vi "Software Update HCC Machine Download Status.vi"(9 "Progam Number":i32, 10 "Station Labels":string[](array[string]), 11 "File Path":path) -> (3 "Status":string)   [LabVIEW 2014]
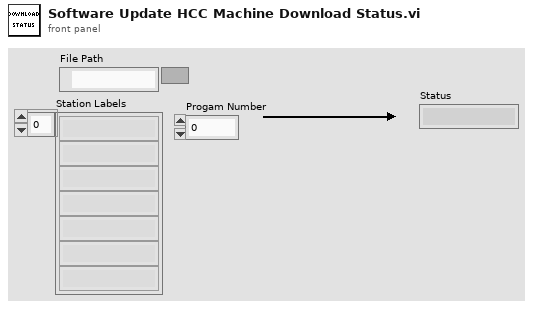
[diagram p1: front panel]
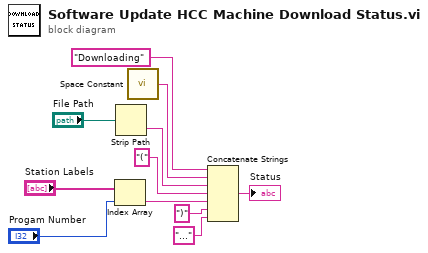
[diagram p0: block diagram]
diagram:
  n1 = Index Array(array="Station Labels", index="Progam Number") -> (element=w10:string)
  n2 = Strip Path(path="File Path") -> (name=w5:string)  [unwired: 1 out]
  n3 = call <vilib>:"Space Constant.vi"() -> ("String"=w3:string)
  n4 = Concatenate Strings("Downloading" ("string"), w3, w5, "(" ("string"), w10, ")" ("string"), "..." ("string")) -> (→"Status":string)
